vi "Finish.vi"   [LabVIEW 2013]
doc: "This VI is called just before exiting. It is expected to close I/O refnum, save collected data, etc."
uses:
  Robot Global Data.vi
  <vilib>/Rock Robotics/WPI/Compressor/WPI_CompressorGetSetRefNum.vi
  <vilib>/Rock Robotics/WPI/RobotDrive/WPI_RobotDriveGetSetRefNum.vi
  <vilib>/Rock Robotics/WPI/Joystick/WPI_JoystickGetSetRefNum.vi
types:
  T1 = typedef "WPI_MotorControlDeviceRef.ctl" = cluster{"DeviceStatus":errorcluster, "Type":enum16{"PWM", "CAN"}, "PWM":cluster{"Digital Module":T2, "PWM Channel":T3, "DeadBand":T4}, "CAN":cluster{"Device Number":u8, "Control Mode":T5, "Semaphore":T6, "Max Vout":dbl}, "Invert":bool, "TransformRef":T7, "InvTransformRef":T7}
  T2 = typedef "FPGA_TypedefDigitalModule.ctl" = enum16{"Digital Module 1", "Digital Module 2"}
  T3 = typedef "FPGA_DIOPWMChannel.ctl" = enum8{"PWM 1", "PWM 2", "PWM 3", "PWM 4", "PWM 5", "PWM 6", "PWM 7", "PWM 8", "PWM 9", "PWM 10", "Invalid"}
  T4 = typedef "WPI_PWMDeadband.ctl" = cluster{"Name":string, "maxPositivePwm":i32, "minPositivePwm":i32, "centerPwm":i32, "maxNegativePwm":i32, "minNegativePwm":i32, "angularRange":u16}
  T5 = typedef "WPI_CANJaguar_ControlMode.ctl" = enum8{"Percent VBus", "Current", "Speed", "Position", "Voltage"}
  T6 = typedef "Semaphore RefNum" = refnum<k1>
  T7 = typedef "WPI_PWMTransform_ConPane.ctl" = refnum<vi>
  T8 = typedef "WPI_SolenoidDevRef.ctl" = cluster{"DevStatus":errorcluster, "Solenoid Module":T9, "Forward Solenoid Channel":T10, "Reverse Solenoid Channel":T10}
  T9 = typedef "FPGA_TypedefSolenoidModule.ctl" = enum16{"Solenoid Module 1", "Solenoid Module 2"}
  T10 = typedef "WPI_SolenoidChannel.ctl" = enum8{"Solenoid 1", "Solenoid 2", "Solenoid 3", "Solenoid 4", "Solenoid 5", "Solenoid 6", "Solenoid 7", "Solenoid 8", "Invalid"}
  T11 = typedef "WPI_RobotDriveDevRef.ctl" = cluster{"DevStatus":errorcluster, "Motors[]":T1[], "Square Inputs":bool, "Max Output":dbl, "Isochronous":bool}
  T12 = typedef "WPI_DigitalInputDevRef.ctl" = cluster{"DevStatus":errorcluster, "DIO Channel":T13, "Digital Module":T2}
  T13 = typedef "FPGA_DIOChannel.ctl" = enum8{"DIO 1", "DIO 2", "DIO 3", "DIO 4", "DIO 5", "DIO 6", "DIO 7", "DIO 8", "DIO 9", "DIO 10", "DIO 11", "DIO 12", "DIO 13", "DIO 14", "Invalid"}
  T14 = typedef "WPI_EncoderDevRef.ctl" = cluster{"DevStatus":errorcluster, "EncoderIndex":T15, "CounterIndex":T16, "DistancePerCount":dbl, "Decoding Type":T17}
  T15 = typedef "FPGA_EncoderIdx.ctl" = enum8{"Enc 0", "Enc 1", "Enc 2", "Enc 3", "Invalid"}
  T16 = typedef "FPGA_CounterCtrSystemIndex.ctl" = enum8{"Ctr 0", "Ctr 1", "Ctr 2", "Ctr 3", "Ctr 4", "Ctr 5", "Ctr 6", "Ctr 7", "Invalid"}
  T17 = typedef "WPI_EncoderType.ctl" = enum16{"1x", "2x", "4x"}
  T18 = typedef "WPI_AnalogChannelDevRef.ctl" = cluster{"DevStatus":errorcluster, "Analog Module":T19, "Analog Channel":T20}
  T19 = typedef "FPGA_TypedefAnalogModule.ctl" = enum16{"Analog Module 1", "Analog Module 2"}
  T20 = typedef "FPGA_AIChannel.ctl" = enum8{"AI 1", "AI 2", "AI 3", "AI 4", "AI 5", "AI 6", "AI 7", "AI 8", "Invalid"}
  T21 = typedef "WPI_CompressorDevRef.ctl" = cluster{"DevStatus":errorcluster, "DigitalInputDevRef":T12, "RelayDevRef":T22}
  T22 = typedef "WPI_RelayDevRef.ctl" = cluster{"DevStatus":errorcluster, "Relay Channel":T23, "Digital Module":T2, "Relay Direction":T24}
  T23 = typedef "FPGA_DIORelayChannel.ctl" = enum8{"Relay 1", "Relay 2", "Relay 3", "Relay 4", "Relay 5", "Relay 6", "Relay 7", "Relay 8", "Invalid"}
  T24 = typedef "WPI_RelayDirection.ctl" = enum16{"Both directions", "Forward only", "Reverse only"}
  T25 = typedef "WPI_ServoDeviceRef.ctl" = cluster{"DeviceStatus":errorcluster, "Digital Module":T2, "PWM Channel":T3, "DeadBand":T4}
  T26 = typedef "WPI_JoystickDevRef.ctl" = cluster{"Device":T27}
  T27 = typedef "WPI_JoystickDeviceEnum.ctl" = enum16{"USB 1", "USB 2", "USB 3", "USB 4", "Kinect 1", "Kinect 2"}
  T28 = typedef "Arcade Drive Ref.ctl" = cluster{"L1":T1, "L2":T1, "R1":T1, "R2":T1, "Motor Count":enum16{"2 Motor", "4 Motor"}, "L Reversed?":bool, "R Reversed?":bool}
  T29 = typedef "WPI_GyroDevRef.ctl" = cluster{"DevStatus":errorcluster, "Analog Module":T19, "Analog Channel":T20, "Offset":dbl, "Gain (VoltsPerDegree/Second)":dbl}
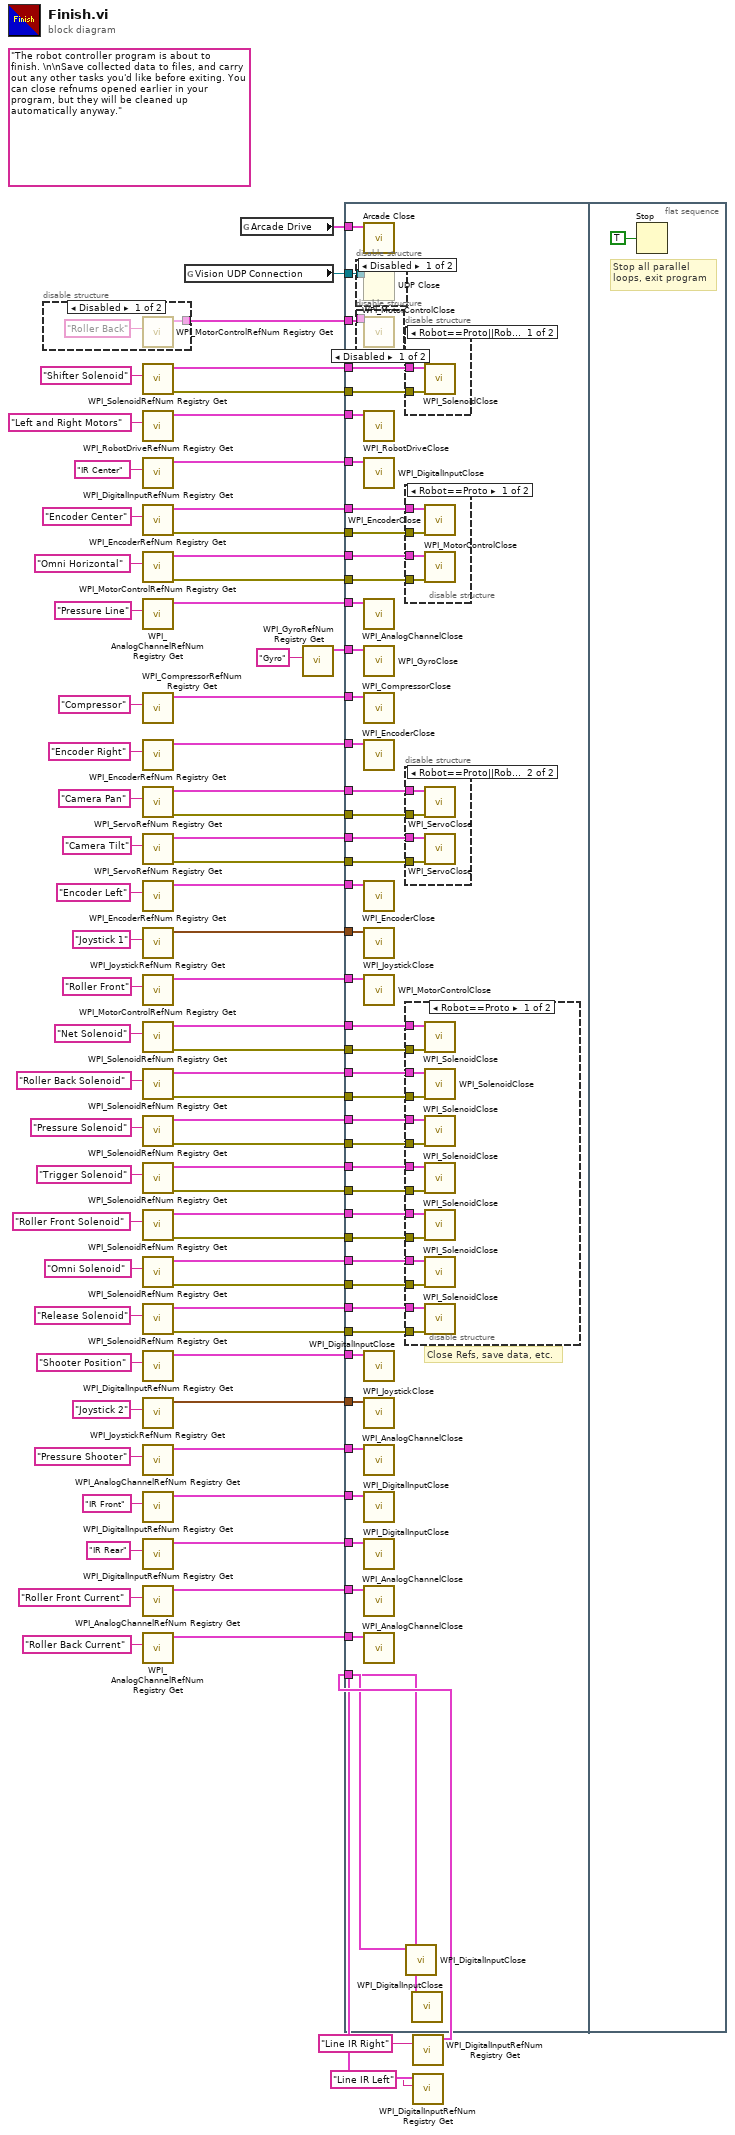
[diagram p0: block diagram]
diagram:
  (unwired) "The robot controller program is about to finish. \n\nSave collected data to files, and carry out any other tasks you'd like before exiting. You can close refnums opened earlier in your program, but they will be cleaned up automatically anyway."
  n1 = disable-structure shown="Disabled" {
    disable-tunnel: [w77 _] -> w55
    frame Disabled {
      n2 = call <vilib>:"WPI_MotorControlRefNum Registry Get.vi"("refnum name"="Roller Back") -> ("MotorControlDevRef"=w77:T1)  [unwired: 9 in, 1 out]
    }
    frame Enabled {
    }
  }
  n3 = call <vilib>:"WPI_SolenoidRefNum Registry Get.vi"("refnum name"="Shifter Solenoid") -> ("error out"=w27:errorcluster, "SolenoidDevRef"=w26:T8)  [unwired: 9 in]
  n4 = call <vilib>:"WPI_RobotDriveRefNum Registry Get.vi"("refnum name"="Left and Right Motors") -> ("RobotDriveDevRef"=w46:T11)  [unwired: 1 in, 9 out]
  n5 = call <vilib>:"WPI_DigitalInputRefNum Registry Get.vi"("refnum name"="IR Center") -> ("DigitalInputDevRef"=w71:T12)  [unwired: 9 in, 1 out]
  n6 = call <vilib>:"WPI_EncoderRefNum Registry Get.vi"("refnum name"="Encoder Center") -> ("error out"=w36:errorcluster, "EncoderDevRef"=w41:T14)  [unwired: 9 in]
  n7 = call <vilib>:"WPI_MotorControlRefNum Registry Get.vi"("refnum name"="Omni Horizontal") -> ("error out"=w35:errorcluster, "MotorControlDevRef"=w34:T1)  [unwired: 9 in]
  n8 = call <vilib>:"WPI_AnalogChannelRefNum Registry Get.vi"("refnum name"="Pressure Line") -> ("AIDeviceRef"=w59:T18)  [unwired: 9 in, 1 out]
  n9 = call <vilib>:"WPI_CompressorRefNum Registry Get.vi"("refnum name"="Compressor") -> ("CompressorDevRef"=w44:T21)  [unwired: 9 in, 1 out]
  n10 = call <vilib>:"WPI_EncoderRefNum Registry Get.vi"("refnum name"="Encoder Right") -> ("EncoderDevRef"=w54:T14)  [unwired: 9 in, 1 out]
  n11 = call <vilib>:"WPI_ServoRefNum Registry Get.vi"("refnum name"="Camera Pan") -> ("error out"=w31:errorcluster, "ServoDeviceRef"=w37:T25)  [unwired: 9 in]
  n12 = call <vilib>:"WPI_ServoRefNum Registry Get.vi"("refnum name"="Camera Tilt") -> ("error out"=w32:errorcluster, "ServoDeviceRef"=w38:T25)  [unwired: 9 in]
  n13 = call <vilib>:"WPI_EncoderRefNum Registry Get.vi"("refnum name"="Encoder Left") -> ("EncoderDevRef"=w52:T14)  [unwired: 9 in, 1 out]
  n14 = call <vilib>:"WPI_JoystickRefNum Registry Get.vi"("refnum name"="Joystick 1") -> ("JoystickDevRef"=w48:T26)  [unwired: 1 in, 9 out]
  n15 = call <vilib>:"WPI_MotorControlRefNum Registry Get.vi"("refnum name"="Roller Front") -> ("MotorControlDevRef"=w57:T1)  [unwired: 9 in, 1 out]
  n16 = call <vilib>:"WPI_SolenoidRefNum Registry Get.vi"("refnum name"="Net Solenoid") -> ("error out"=w9:errorcluster, "SolenoidDevRef"=w8:T8)  [unwired: 9 in]
  n17 = call <vilib>:"WPI_SolenoidRefNum Registry Get.vi"("refnum name"="Roller Back Solenoid") -> ("error out"=w12:errorcluster, "SolenoidDevRef"=w11:T8)  [unwired: 9 in]
  n18 = call <vilib>:"WPI_SolenoidRefNum Registry Get.vi"("refnum name"="Pressure Solenoid") -> ("error out"=w24:errorcluster, "SolenoidDevRef"=w23:T8)  [unwired: 9 in]
  n19 = call <vilib>:"WPI_SolenoidRefNum Registry Get.vi"("refnum name"="Trigger Solenoid") -> ("error out"=w21:errorcluster, "SolenoidDevRef"=w20:T8)  [unwired: 9 in]
  n20 = call <vilib>:"WPI_SolenoidRefNum Registry Get.vi"("refnum name"="Roller Front Solenoid") -> ("error out"=w15:errorcluster, "SolenoidDevRef"=w14:T8)  [unwired: 9 in]
  n21 = call <vilib>:"WPI_SolenoidRefNum Registry Get.vi"("refnum name"="Omni Solenoid") -> ("error out"=w30:errorcluster, "SolenoidDevRef"=w29:T8)  [unwired: 9 in]
  n22 = call <vilib>:"WPI_SolenoidRefNum Registry Get.vi"("refnum name"="Release Solenoid") -> ("error out"=w18:errorcluster, "SolenoidDevRef"=w17:T8)  [unwired: 9 in]
  n23 = call <vilib>:"WPI_DigitalInputRefNum Registry Get.vi"("refnum name"="Shooter Position") -> ("DigitalInputDevRef"=w63:T12)  [unwired: 9 in, 1 out]
  n24 = call <vilib>:"WPI_JoystickRefNum Registry Get.vi"("refnum name"="Joystick 2") -> ("JoystickDevRef"=w50:T26)  [unwired: 9 in, 1 out]
  n25 = call <vilib>:"WPI_AnalogChannelRefNum Registry Get.vi"("refnum name"="Pressure Shooter") -> ("AIDeviceRef"=w65:T18)  [unwired: 9 in, 1 out]
  n26 = call <vilib>:"WPI_DigitalInputRefNum Registry Get.vi"("refnum name"="IR Front") -> ("DigitalInputDevRef"=w67:T12)  [unwired: 9 in, 1 out]
  n27 = call <vilib>:"WPI_DigitalInputRefNum Registry Get.vi"("refnum name"="IR Rear") -> ("DigitalInputDevRef"=w69:T12)  [unwired: 9 in, 1 out]
  n28 = call <vilib>:"WPI_AnalogChannelRefNum Registry Get.vi"("refnum name"="Roller Front Current") -> ("AIDeviceRef"=w73:T18)  [unwired: 9 in, 1 out]
  n29 = call <vilib>:"WPI_AnalogChannelRefNum Registry Get.vi"("refnum name"="Roller Back Current") -> ("AIDeviceRef"=w75:T18)  [unwired: 9 in, 1 out]
  n30 = global read "Robot Global Data.vi" "Vision UDP Connection"() -> (w6:refnum<k16>)
  n31 = global read "Robot Global Data.vi" "Arcade Drive"() -> (w5:T28)
  n32 = call <vilib>:"WPI_GyroRefNum Registry Get.vi"("refnum name"="Gyro") -> ("GyroDevRef"=w61:T29)  [unwired: 9 in, 1 out]
  n33 = flat-sequence {
    tunnel: w75 -> [w122]
    tunnel: w73 -> [w121]
    tunnel: w71 -> [w120]
    tunnel: w69 -> [w119]
    tunnel: w67 -> [w118]
    tunnel: w65 -> [w117]
    tunnel: w63 -> [w116]
    tunnel: w18 -> [w87]
    tunnel: w30 -> [w94]
    tunnel: w61 -> [w115]
    tunnel: w29 -> [w95]
    tunnel: w6 -> [w114]
    tunnel: w15 -> [w85]
    tunnel: w59 -> [w113]
    tunnel: w35 -> [w102]
    tunnel: w57 -> [w112]
    tunnel: w55 -> [w111]
    tunnel: w21 -> [w89]
    tunnel: w54 -> [w103]
    tunnel: w52 -> [w101]
    tunnel: w50 -> [w110]
    tunnel: w48 -> [w109]
    tunnel: w46 -> [w108]
    tunnel: w44 -> [w107]
    tunnel: w26 -> [w93]
    tunnel: w27 -> [w92]
    tunnel: w24 -> [w91]
    tunnel: w5 -> [w106]
    tunnel: w41 -> [w105]
    tunnel: w38 -> [w98]
    tunnel: w37 -> [w97]
    tunnel: w36 -> [w104]
    tunnel: w34 -> [w100]
    tunnel: w32 -> [w99]
    tunnel: w31 -> [w96]
    tunnel: w23 -> [w90]
    tunnel: w20 -> [w88]
    tunnel: w17 -> [w86]
    tunnel: w14 -> [w84]
    tunnel: w12 -> [w83]
    tunnel: w11 -> [w82]
    tunnel: w8 -> [w81]
    tunnel: w9 -> [w80]
    tunnel: w4 -> [w79]
    tunnel: w2 -> [w78]
    frame #0 {
      # "Close Refs, save data, etc."
      n34 = disable-structure shown="Disabled" {
        disable-tunnel: w114 -> [w124 _]
        frame Disabled {
          n35 = UDP Close(connection ID=w124) -> ()  [unwired: 1 in, 2 out]
        }
        frame Enabled {
        }
      }
      n36 = disable-structure shown="Disabled" {
        disable-tunnel: w111 -> [w123 _]
        frame Disabled {
          n37 = call <vilib>:"WPI_MotorControlClose.vi"("MotorControlDevRef"=w123) -> ()  [unwired: 10 in, 1 out]
        }
        frame Enabled {
        }
      }
      n38 = call "Arcade Close.vi"("output cluster"=w106) -> ()  [unwired: 11 in]
      n39 = call <vilib>:"WPI_RobotDriveClose.vi"("RobotDriveDevRef"=w108) -> ()  [unwired: 1 in, 10 out]
      n40 = call <vilib>:"WPI_DigitalInputClose.vi"("DigitalInputDevRef"=w120) -> ()  [unwired: 10 in, 1 out]
      n41 = call <vilib>:"WPI_AnalogChannelClose.vi"("AIDeviceRef"=w113) -> ()  [unwired: 10 in, 1 out]
      n42 = call <vilib>:"WPI_GyroClose.vi"("GyroDevRef"=w115) -> ()  [unwired: 10 in, 1 out]
      n43 = call <vilib>:"WPI_CompressorClose.vi"("CompressorDevRef"=w107) -> ()  [unwired: 10 in, 1 out]
      n44 = call <vilib>:"WPI_EncoderClose.vi"("EncoderDevRef"=w103) -> ()  [unwired: 10 in, 1 out]
      n45 = call <vilib>:"WPI_EncoderClose.vi"("EncoderDevRef"=w101) -> ()  [unwired: 10 in, 1 out]
      n46 = call <vilib>:"WPI_JoystickClose.vi"("JoystickDevRef"=w109) -> ()  [unwired: 11 out]
      n47 = call <vilib>:"WPI_MotorControlClose.vi"("MotorControlDevRef"=w112) -> ()  [unwired: 10 in, 1 out]
      n48 = call <vilib>:"WPI_DigitalInputClose.vi"("DigitalInputDevRef"=w116) -> ()  [unwired: 10 in, 1 out]
      n49 = call <vilib>:"WPI_JoystickClose.vi"("JoystickDevRef"=w110) -> ()  [unwired: 11 out]
      n50 = call <vilib>:"WPI_AnalogChannelClose.vi"("AIDeviceRef"=w117) -> ()  [unwired: 10 in, 1 out]
      n51 = call <vilib>:"WPI_DigitalInputClose.vi"("DigitalInputDevRef"=w118) -> ()  [unwired: 10 in, 1 out]
      n52 = call <vilib>:"WPI_DigitalInputClose.vi"("DigitalInputDevRef"=w119) -> ()  [unwired: 10 in, 1 out]
      n53 = call <vilib>:"WPI_AnalogChannelClose.vi"("AIDeviceRef"=w121) -> ()  [unwired: 10 in, 1 out]
      n54 = call <vilib>:"WPI_AnalogChannelClose.vi"("AIDeviceRef"=w122) -> ()  [unwired: 10 in, 1 out]
      n55 = disable-structure shown="Robot==Proto||Robot==Frogger" {
        disable-tunnel: w93 -> [w125 _]
        disable-tunnel: w92 -> [w126 _]
        frame condition #0 (active) {
          n56 = call <vilib>:"WPI_SolenoidClose.vi"("error in (no error)"=w126, "SolenoidDevRef"=w125) -> ()  [unwired: 9 in, 1 out]
        }
        frame condition #1 {
        }
      }
      n57 = disable-structure shown="Robot==Proto" {
        disable-tunnel: w104 -> [w147 _]
        disable-tunnel: w102 -> [w146 _]
        disable-tunnel: w105 -> [w148 _]
        disable-tunnel: w100 -> [w145 _]
        frame condition #0 (active) {
          n58 = call <vilib>:"WPI_EncoderClose.vi"("error in (no error)"=w147, "EncoderDevRef"=w148) -> ()  [unwired: 9 in, 1 out]
          n59 = call <vilib>:"WPI_MotorControlClose.vi"("error in (no error)"=w146, "MotorControlDevRef"=w145) -> ()  [unwired: 9 in, 1 out]
        }
        frame condition #1 {
        }
      }
      n60 = disable-structure shown="Robot==Proto||Robot==Whiplash" {
        disable-tunnel: w97 -> [_ w142]
        disable-tunnel: w96 -> [_ w141]
        disable-tunnel: w98 -> [_ w144]
        disable-tunnel: w99 -> [_ w143]
        frame condition #0 {
        }
        frame condition #1 (active) {
          n61 = call <vilib>:"WPI_ServoClose.vi"("error in (no error)"=w141, "MotorControlDevRef"=w142) -> ()  [unwired: 9 in, 1 out]
          n62 = call <vilib>:"WPI_ServoClose.vi"("error in (no error)"=w143, "MotorControlDevRef"=w144) -> ()  [unwired: 9 in, 1 out]
        }
      }
      n63 = disable-structure shown="Robot==Proto" {
        disable-tunnel: w90 -> [w140 _]
        disable-tunnel: w86 -> [w136 _]
        disable-tunnel: w84 -> [w139 _]
        disable-tunnel: w88 -> [w133 _]
        disable-tunnel: w82 -> [w138 _]
        disable-tunnel: w95 -> [w127 _]
        disable-tunnel: w81 -> [w129 _]
        disable-tunnel: w94 -> [w132 _]
        disable-tunnel: w85 -> [w130 _]
        disable-tunnel: w87 -> [w134 _]
        disable-tunnel: w89 -> [w131 _]
        disable-tunnel: w91 -> [w128 _]
        disable-tunnel: w83 -> [w137 _]
        disable-tunnel: w80 -> [w135 _]
        frame condition #0 (active) {
          n64 = call <vilib>:"WPI_SolenoidClose.vi"("error in (no error)"=w135, "SolenoidDevRef"=w129) -> ()  [unwired: 9 in, 1 out]
          n65 = call <vilib>:"WPI_SolenoidClose.vi"("error in (no error)"=w137, "SolenoidDevRef"=w138) -> ()  [unwired: 9 in, 1 out]
          n66 = call <vilib>:"WPI_SolenoidClose.vi"("error in (no error)"=w128, "SolenoidDevRef"=w140) -> ()  [unwired: 9 in, 1 out]
          n67 = call <vilib>:"WPI_SolenoidClose.vi"("error in (no error)"=w131, "SolenoidDevRef"=w133) -> ()  [unwired: 9 in, 1 out]
          n68 = call <vilib>:"WPI_SolenoidClose.vi"("error in (no error)"=w130, "SolenoidDevRef"=w139) -> ()  [unwired: 9 in, 1 out]
          n69 = call <vilib>:"WPI_SolenoidClose.vi"("error in (no error)"=w132, "SolenoidDevRef"=w127) -> ()  [unwired: 9 in, 1 out]
          n70 = call <vilib>:"WPI_SolenoidClose.vi"("error in (no error)"=w134, "SolenoidDevRef"=w136) -> ()  [unwired: 9 in, 1 out]
        }
        frame condition #1 {
        }
      }
      n71 = call <vilib>:"WPI_DigitalInputClose.vi"("DigitalInputDevRef"=w79) -> ()  [unwired: 10 in, 1 out]
      n72 = call <vilib>:"WPI_DigitalInputClose.vi"("DigitalInputDevRef"=w78) -> ()  [unwired: 10 in, 1 out]
    }
    frame #1 {
      # "Stop all parallel\nloops, exit program"
      n73 = Stop(stop? (T)=TRUE ("Quit")) -> ()
    }
  }
  n74 = call <vilib>:"WPI_DigitalInputRefNum Registry Get.vi"("refnum name"="Line IR Right") -> ("DigitalInputDevRef"=w4:T12)  [unwired: 9 in, 1 out]
  n75 = call <vilib>:"WPI_DigitalInputRefNum Registry Get.vi"("refnum name"="Line IR Left") -> ("DigitalInputDevRef"=w2:T12)  [unwired: 9 in, 1 out]
